vi "Panel to Screen Cords Converter.vi"(6 "VI Ref":refnum<vi>, 8 "Vertical FP 2":i32, 9 "Vertical FP 1":i32, 10 "Horizontal FP 2":i32, 11 "Horizontal FP 1":i32) -> (0 "Vertical Screen 2":i16, 1 "Vertical Screen 1":i16, 2 "Horizontal Screen 2":i16, 3 "Horizontal Screen 1":i16)   [LabVIEW 2016]
uses:
  <vilib>/Utility/miscctls.llb/LVPointTypeDef.ctl
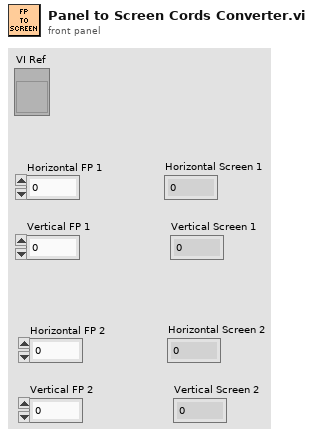
[diagram p1: front panel]
types:
  T1 = typedef "LVPointTypeDef.ctl" = cluster{"Horizontal":i16, "Vertical":i16}
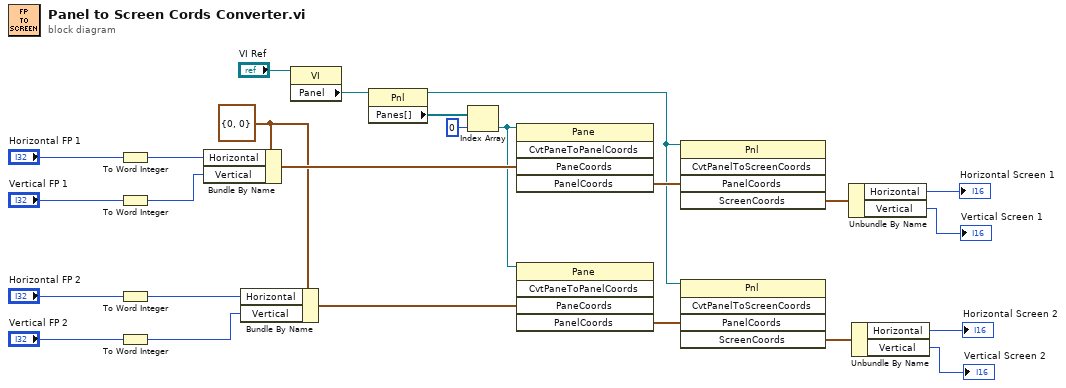
[diagram p0: block diagram]
diagram:
  w7 = T1 {"Horizontal"=0, "Vertical"=0} ("Pane Coordinates")
  n1 = To Word Integer(number="Horizontal FP 1") -> (16bit integer=w4:i16)
  n2 = To Word Integer(number="Vertical FP 1") -> (16bit integer=w3:i16)
  n3 = To Word Integer(number="Horizontal FP 2") -> (16bit integer=w2:i16)
  n4 = To Word Integer(number="Vertical FP 2") -> (16bit integer=w1:i16)
  n5 = Bundle By Name(cluster=w7, "Horizontal"=w4, "Vertical"=w3) -> (w18:T1)
  n6 = Bundle By Name(cluster=w7, "Horizontal"=w2, "Vertical"=w1) -> (w11:T1)
  n7 = property class="VI"(reference="VI Ref") -> ("Panel"=w23:refnum<vi>)  [unwired: 1 in, 2 out]
  n8 = property class="Pnl"(reference=w23) -> (reference out=w5:refnum<vi>, "Panes[]"=w25:refnum<vi>[])  [unwired: 1 in, 1 out]
  n9 = Index Array(array=w25, index=0) -> (element=w6:refnum<vi>)
  n10 = invoke class="Pane" method="CvtPaneToPanelCoords"(reference=w6, "PaneCoords"=w18) -> ("PanelCoords"=w22:T1)  [unwired: 3 in, 4 out]
  n11 = invoke class="Pane" method="CvtPaneToPanelCoords"(reference=w6, "PaneCoords"=w11) -> ("PanelCoords"=w8:T1)  [unwired: 3 in, 4 out]
  n12 = invoke class="Pnl" method="CvtPanelToScreenCoords"(reference=w5, "PanelCoords"=w22) -> ("ScreenCoords"=w17:T1)  [unwired: 3 in, 4 out]
  n13 = invoke class="Pnl" method="CvtPanelToScreenCoords"(reference=w5, "PanelCoords"=w8) -> ("ScreenCoords"=w12:T1)  [unwired: 3 in, 4 out]
  n14 = Unbundle By Name(w17) -> ("Horizontal"=→"Horizontal Screen 1":i16, "Vertical"=→"Vertical Screen 1":i16)
  n15 = Unbundle By Name(w12) -> ("Horizontal"=→"Horizontal Screen 2":i16, "Vertical"=→"Vertical Screen 2":i16)
